vi "PXI4072 Initialize.vi"(8 "error in (no error)":errorcluster, 11 "PXI4072 All UI Refs":T1) -> (0 "error out":errorcluster)   [LabVIEW 2026]
uses:
  App Types/References/PXI4072 All UI References.ctl
  App Types/References/PXI4072 Boolean UI References.ctl
  App Types/References/PXI4072 String UI References.ctl
  App Types/References/PXI4072 Numeric UI References.ctl
  App Types/References/PXI4072 Other UI Rerences.ctl
  Drivers/PXI4072/Types/PXI4072 Settings.ctl
  <instrlib>/niDMM/nidmm.llb/niDMM Function.ctl
  <instrlib>/niDMM/nidmm.llb/niDMM Resolution in Digits.ctl
  Drivers/PXI4072/PXI4072.lvlib
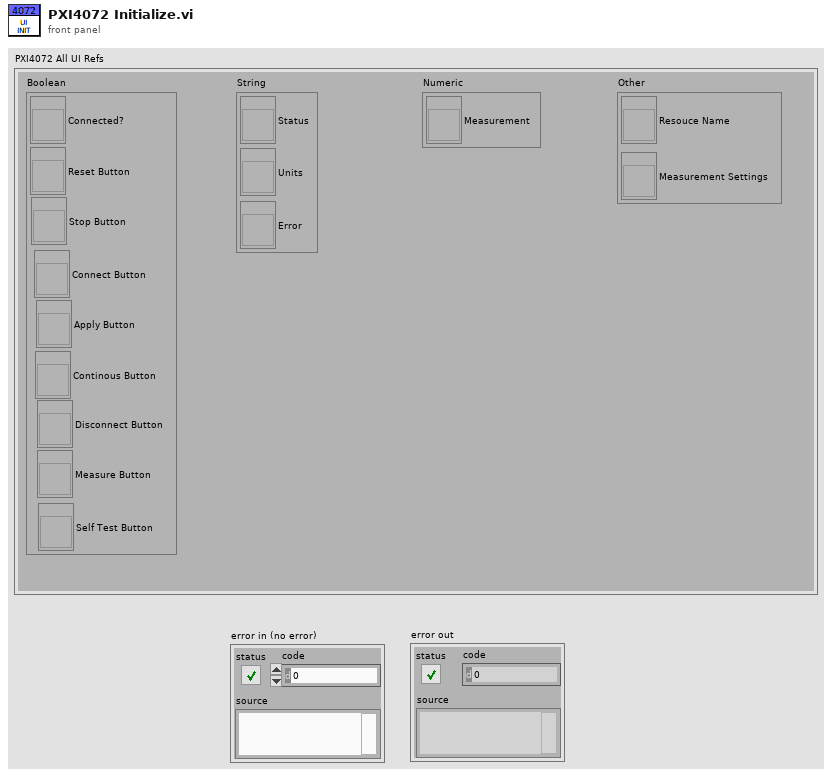
[diagram p1: front panel]
types:
  T1 = typedef "PXI4072 All UI References.ctl" = cluster{"Boolean":T2, "String":T3, "Numeric":T4, "Other":T5}
  T2 = typedef "PXI4072 Boolean UI References.ctl" = cluster{"Connected?":refnum<vi>, "Reset Button":refnum<vi>, "Connect Button":refnum<vi>, "Apply Button":refnum<vi>, "Disconnect Button":refnum<vi>, "Measure Button":refnum<vi>, "Self Test Button":refnum<vi>, "Continous Button":refnum<vi>, "Stop Button":refnum<vi>}
  T3 = typedef "PXI4072 String UI References.ctl" = cluster{"Status":refnum<vi>, "Units":refnum<vi>, "Error":refnum<vi>}
  T4 = typedef "PXI4072 Numeric UI References.ctl" = cluster{"Measurement":refnum<vi>}
  T5 = typedef "PXI4072 Other UI Rerences.ctl" = cluster{"Resouce Name":refnum<vi>, "Measurement Settings":refnum<vi>}
  T6 = enum8{"Enabled", "Disabled", "Disabled and Grayed Out"}
  T7 = typedef "PXI4072.lvlib/PXI4072 Settings.ctl" = cluster{"Function":T8, "Resolution in Digits":T9, "Range":dbl}
  T8 = typedef "niDMM Function.ctl" = enum16{"DC Volts", "AC Volts", "DC Current", "AC Current", "2-wire Resistance", "4-wire Resistance", "Diode", "Frequency", "Period", "AC Volts DC Coupled", "Capacitance", "Inductance", "Temperature"}
  T9 = typedef "niDMM Resolution in Digits.ctl" = dbl
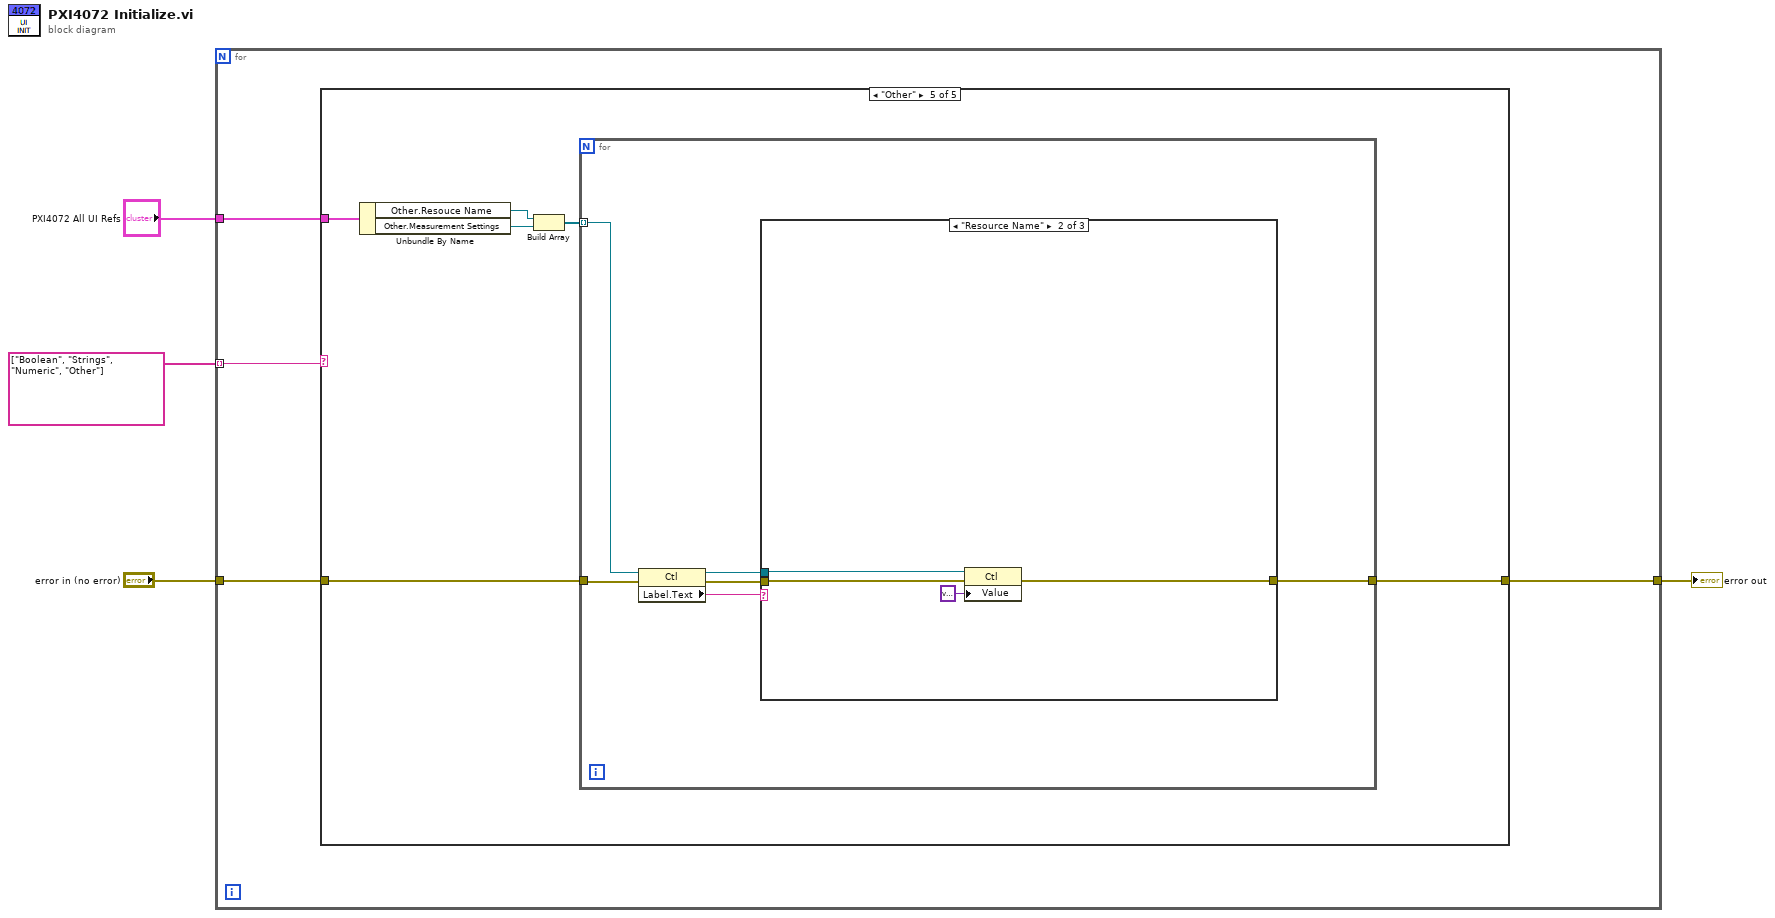
[diagram p0: block diagram]
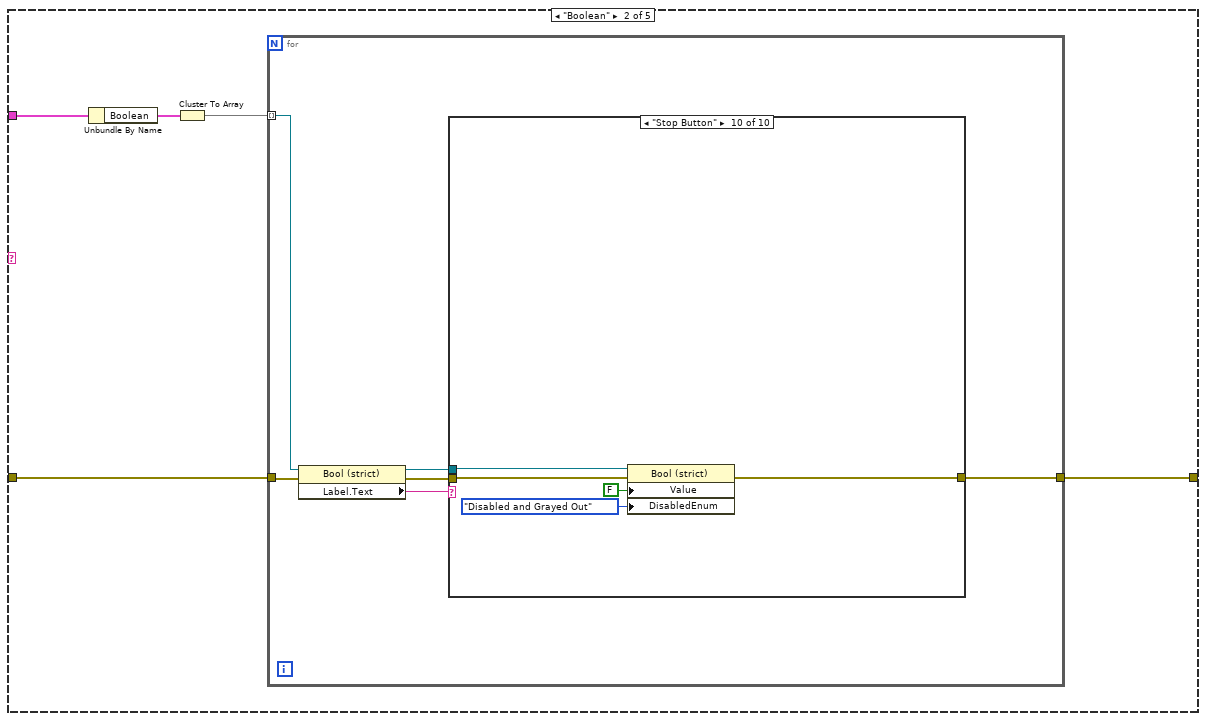
[diagram p3: hidden frame]
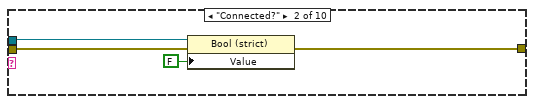
[diagram p5: hidden frame]
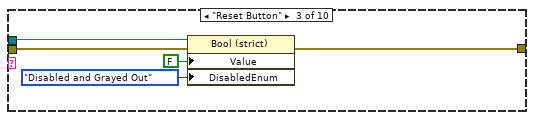
[diagram p6: hidden frame]
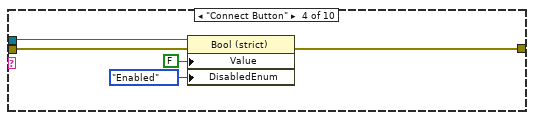
[diagram p7: hidden frame]
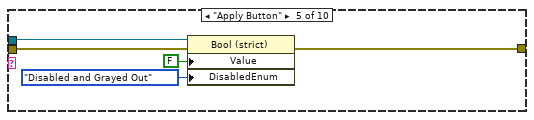
[diagram p8: hidden frame]
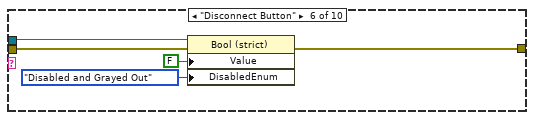
[diagram p9: hidden frame]
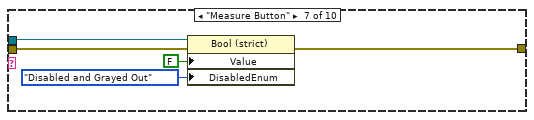
[diagram p10: hidden frame]
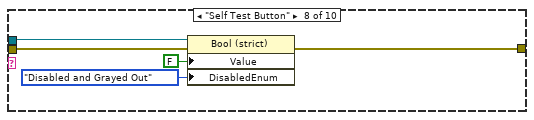
[diagram p11: hidden frame]
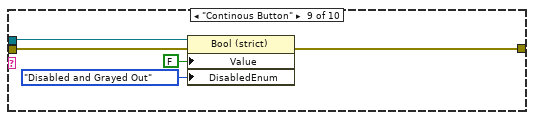
[diagram p12: hidden frame]
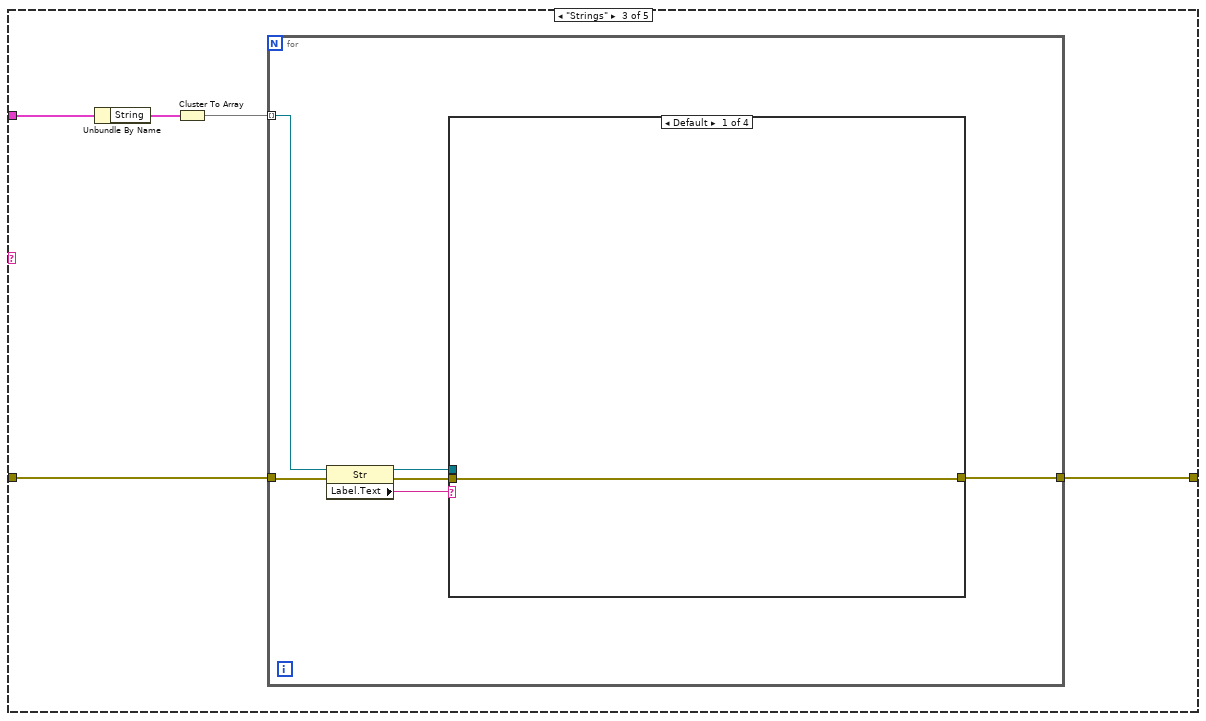
[diagram p13: hidden frame]
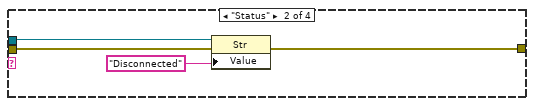
[diagram p14: hidden frame]
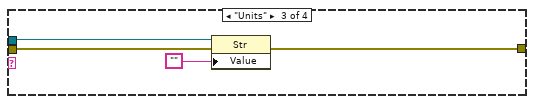
[diagram p15: hidden frame]
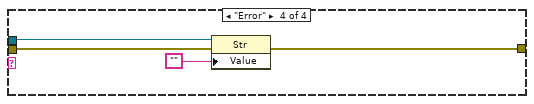
[diagram p16: hidden frame]
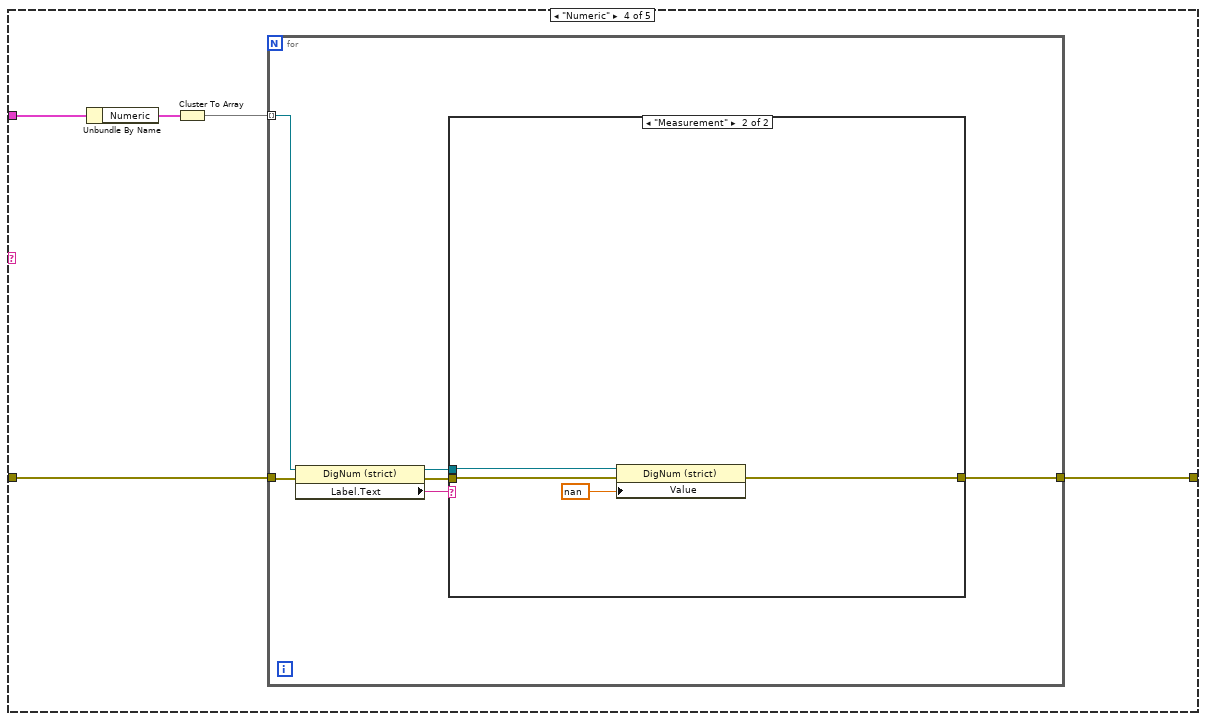
[diagram p17: hidden frame]
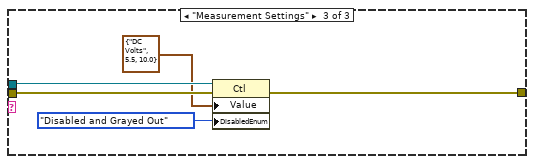
[diagram p20: hidden frame]
diagram:
  n1 = for {
    tunnel: string[] ["Boolean", "Strings", "Numeric", "Other"] -> [w8] mode=indexing
    tunnel: "PXI4072 All UI Refs" -> [w7]
    tunnel: "error in (no error)" -> [w6]
    tunnel: [w5] -> w2
    n2 = case shown="\"Other\"" w8 {
      tunnel: w7 -> [_ w14 w70 w94 w111]
      tunnel: w6 -> [w9 w11 w67 w91 w110]
      tunnel: [w9 w10 w66 w90 w109] -> w5
      frame Default {
      }
      frame "Boolean" {
        n3 = Unbundle By Name(w14) -> ("Boolean"=w13:T2)
        n4 = Cluster To Array(cluster=w13) -> (array=w12:refnum<vi>[])
        n5 = for {
          tunnel: w12 -> [w19] mode=indexing
          tunnel: w11 -> [w20]
          tunnel: [w15] -> w10
          n6 = property class="Bool (strict)"(reference=w19, error in=w20) -> (reference out=w16:refnum<vi>, error out=w18:errorcluster, "Label.Text"=w17:string)
          n7 = case shown="\"Stop Button\"" w17 {
            tunnel: w18 -> [w21 w25 w30 w35 w40 w45 w50 w55 w60 w65]
            tunnel: w16 -> [_ w23 w28 w33 w38 w43 w48 w53 w58 w63]
            tunnel: [w21 w24 w29 w34 w39 w44 w49 w54 w59 w64] -> w15
            frame Default {
            }
            frame "Connected?" {
              n8 = property class="Bool (strict)"(reference=w23, error in=w25, "Value"=FALSE) -> (error out=w24:errorcluster)  [unwired: 1 out]
            }
            frame "Reset Button" {
              n9 = property class="Bool (strict)"(reference=w28, error in=w30, "Value"=FALSE, "DisabledEnum"=T6."Disabled and Grayed Out" ("Disabled")) -> (error out=w29:errorcluster)  [unwired: 1 out]
            }
            frame "Connect Button" {
              n10 = property class="Bool (strict)"(reference=w33, error in=w35, "Value"=FALSE, "DisabledEnum"=T6."Enabled" ("Disabled")) -> (error out=w34:errorcluster)  [unwired: 1 out]
            }
            frame "Apply Button" {
              n11 = property class="Bool (strict)"(reference=w38, error in=w40, "Value"=FALSE, "DisabledEnum"=T6."Disabled and Grayed Out" ("Disabled")) -> (error out=w39:errorcluster)  [unwired: 1 out]
            }
            frame "Disconnect Button" {
              n12 = property class="Bool (strict)"(reference=w43, error in=w45, "Value"=FALSE, "DisabledEnum"=T6."Disabled and Grayed Out" ("Disabled")) -> (error out=w44:errorcluster)  [unwired: 1 out]
            }
            frame "Measure Button" {
              n13 = property class="Bool (strict)"(reference=w48, error in=w50, "Value"=FALSE, "DisabledEnum"=T6."Disabled and Grayed Out" ("Disabled")) -> (error out=w49:errorcluster)  [unwired: 1 out]
            }
            frame "Self Test Button" {
              n14 = property class="Bool (strict)"(reference=w53, error in=w55, "Value"=FALSE, "DisabledEnum"=T6."Disabled and Grayed Out" ("Disabled")) -> (error out=w54:errorcluster)  [unwired: 1 out]
            }
            frame "Continous Button" {
              n15 = property class="Bool (strict)"(reference=w58, error in=w60, "Value"=FALSE, "DisabledEnum"=T6."Disabled and Grayed Out" ("Disabled")) -> (error out=w59:errorcluster)  [unwired: 1 out]
            }
            frame "Stop Button" {
              n16 = property class="Bool (strict)"(reference=w63, error in=w65, "Value"=FALSE, "DisabledEnum"=T6."Disabled and Grayed Out" ("Disabled")) -> (error out=w64:errorcluster)  [unwired: 1 out]
            }
          }
        }
      }
      frame "Strings" {
        n17 = Unbundle By Name(w70) -> ("String"=w69:T3)
        n18 = Cluster To Array(cluster=w69) -> (array=w68:refnum<vi>[])
        n19 = for {
          tunnel: w68 -> [w75] mode=indexing
          tunnel: w67 -> [w76]
          tunnel: [w71] -> w66
          n20 = property class="Str"(reference=w75, error in=w76) -> (reference out=w72:refnum<vi>, error out=w74:errorcluster, "Label.Text"=w73:string)
          n21 = case shown="Default" w73 {
            tunnel: w74 -> [w77 w81 w85 w89]
            tunnel: w72 -> [_ w79 w83 w87]
            tunnel: [w77 w80 w84 w88] -> w71
            frame Default {
            }
            frame "Status" {
              n22 = property class="Str"(reference=w79, error in=w81, "Value"="Disconnected") -> (error out=w80:errorcluster)  [unwired: 1 out]
            }
            frame "Units" {
              n23 = property class="Str"(reference=w83, error in=w85, "Value"="") -> (error out=w84:errorcluster)  [unwired: 1 out]
            }
            frame "Error" {
              n24 = property class="Str"(reference=w87, error in=w89, "Value"="") -> (error out=w88:errorcluster)  [unwired: 1 out]
            }
          }
        }
      }
      frame "Numeric" {
        n25 = Unbundle By Name(w94) -> ("Numeric"=w93:T4)
        n26 = Cluster To Array(cluster=w93) -> (array=w92:refnum<vi>[])
        n27 = for {
          tunnel: w92 -> [w99] mode=indexing
          tunnel: w91 -> [w100]
          tunnel: [w95] -> w90
          n28 = property class="DigNum (strict)"(reference=w99, error in=w100) -> (reference out=w96:refnum<vi>, error out=w98:errorcluster, "Label.Text"=w97:string)
          n29 = case shown="\"Measurement\"" w97 {
            tunnel: w98 -> [w101 w105]
            tunnel: w96 -> [_ w103]
            tunnel: [w101 w104] -> w95
            frame Default {
            }
            frame "Measurement" {
              n30 = property class="DigNum (strict)"(reference=w103, error in=w105, "Value"=nan) -> (error out=w104:errorcluster)  [unwired: 1 out]
            }
          }
        }
      }
      frame "Other" {
        n31 = Unbundle By Name(w111) -> ("Other.Resouce Name"=w108:refnum<vi>, "Other.Measurement Settings"=w107:refnum<vi>)
        n32 = Build Array(w108, w107) -> (w106:refnum<vi>[])
        n33 = for {
          tunnel: w110 -> [w117]
          tunnel: [w113] -> w109
          tunnel: w106 -> [w112] mode=indexing
          n34 = property class="Ctl"(reference=w112, error in=w117) -> (reference out=w114:refnum<vi>, error out=w116:errorcluster, "Label.Text"=w115:string)
          n35 = case shown="\"Resource Name\"" w115 {
            tunnel: w116 -> [w118 w122 w127]
            tunnel: w114 -> [_ w120 w125]
            tunnel: [w118 w121 w126] -> w113
            frame Default {
            }
            frame "Resource Name" {
              n36 = property class="Ctl"(reference=w120, error in=w122, "Value"=variant) -> (error out=w121:errorcluster)  [unwired: 1 out]
            }
            frame "Measurement Settings" {
              n37 = property class="Ctl"(reference=w125, error in=w127, "Value"=T7 {"Function"=enum."DC Volts", "Resolution in Digits"=5.5, "Range"=10.0} ("Measurement Settings"), "DisabledEnum"=T6."Disabled and Grayed Out" ("Disabled")) -> (error out=w126:errorcluster)  [unwired: 1 out]
            }
          }
        }
      }
    }
  }
  "error out" <- w2
